vi "LaserMarked_ProjectSetPanel.vi"(11 "SetPanelRef":refnum<vi>) -> ()   [LabVIEW 2019]
uses:
  <vilib>/Utility/miscctls.llb/LVPointTypeDef.ctl
  <vilib>/Utility/miscctls.llb/LVPositionTypeDef.ctl
panel:
  out "$Read Project Recipe 2":path=path "C:/Users/MyUser/Desktop/S2_Project.txt" caption="讀取專案名稱路徑"
  in  "$Standar VNum_":string caption="電壓上限"
  in  "$NGY":i32 caption="料盤陣列Y" min=0 step=1
  in  "$NGX":i32 caption="料盤陣列X" min=0 step=1
  in  "$AIY":i32 caption="料盤AI拍照Y方向次數" min=0 step=1
  in  "$AIX":i32 caption="料盤AI拍照X方向次數" min=0 step=1
  in  "$LSY":i32 caption="料盤線掃瞄Y方向次數" min=0 step=1
  in  "$LSX":i32 caption="料盤線掃瞄X方向次數" min=0 step=1
  in  "$VISA resource name":refnum<visa-resource-name>
  in  "$VType":enum16{"無條件捨去", "四捨五入"}(ring) caption="電壓選取方式"
  in  "$Ring":u16(ring) caption="Ring" items=["A", "V", "C"]
  in  "Tab Control":enum32{"Page 1", "Page 2"}(tab)
  in  "$PLC_First PD No":i32 caption="PLC 使用首件號碼" min=0 step=1
  in  "$Read Tool Initial Project":path=path "C:/Users/MyUser/Desktop/S2_Project.txt" caption="讀取Tool Initial專案"
  in  "$Read S4 Tool Project":path=path "C:/Users/MyUser/Desktop/S2_Project.txt" caption="讀取S4 Tool專案路徑"
  in  "$Read S3 Tool Project":path=path "C:/Users/MyUser/Desktop/S2_Project.txt" caption="讀取S3 Tool專案路徑"
  in  "$Read S2 Tool Project":path=path "C:/Users/MyUser/Desktop/S2_Project.txt" caption="讀取S2 Tool專案路徑"
  in  "$RSSI Dn":dbl caption="RSSI下限" format="%#_13g"
  in  "$RSSI Up":dbl caption="RSSI上限" format="%#_13g"
  in  "$V Dn":dbl caption="V下限" format="%#_13g"
  in  "$C Dn":dbl caption="C(溫度值)下限" format="%#_13g"
  in  "$C Up":dbl caption="C(溫度值上限)" format="%#_13g"
  in  "$V Up":dbl caption="V 上限" format="%#_13g"
  in  "$MeasurLow":dbl caption="測高下限" format="%#_13g"
  in  "$MeasurHigh":dbl caption="測高上限" format="%#_13g"
  in  "$Current Dn":dbl caption="電流下限" format="%#_13g"
  in  "$Voltage Dn":dbl caption="電壓下限" format="%#_13g"
  in  "$ForceSetBinChk_":bool caption="使用參數確認"
  in  "$Voltage Up":dbl caption="電壓上限" format="%#_13g"
  in  "$Current Up":dbl caption="電流上限" format="%#_13g"
  in  "$PLC_Project No":i32 caption="PLC 使用專案號碼" min=0 step=1
  # "藍芽檢查參數設定"
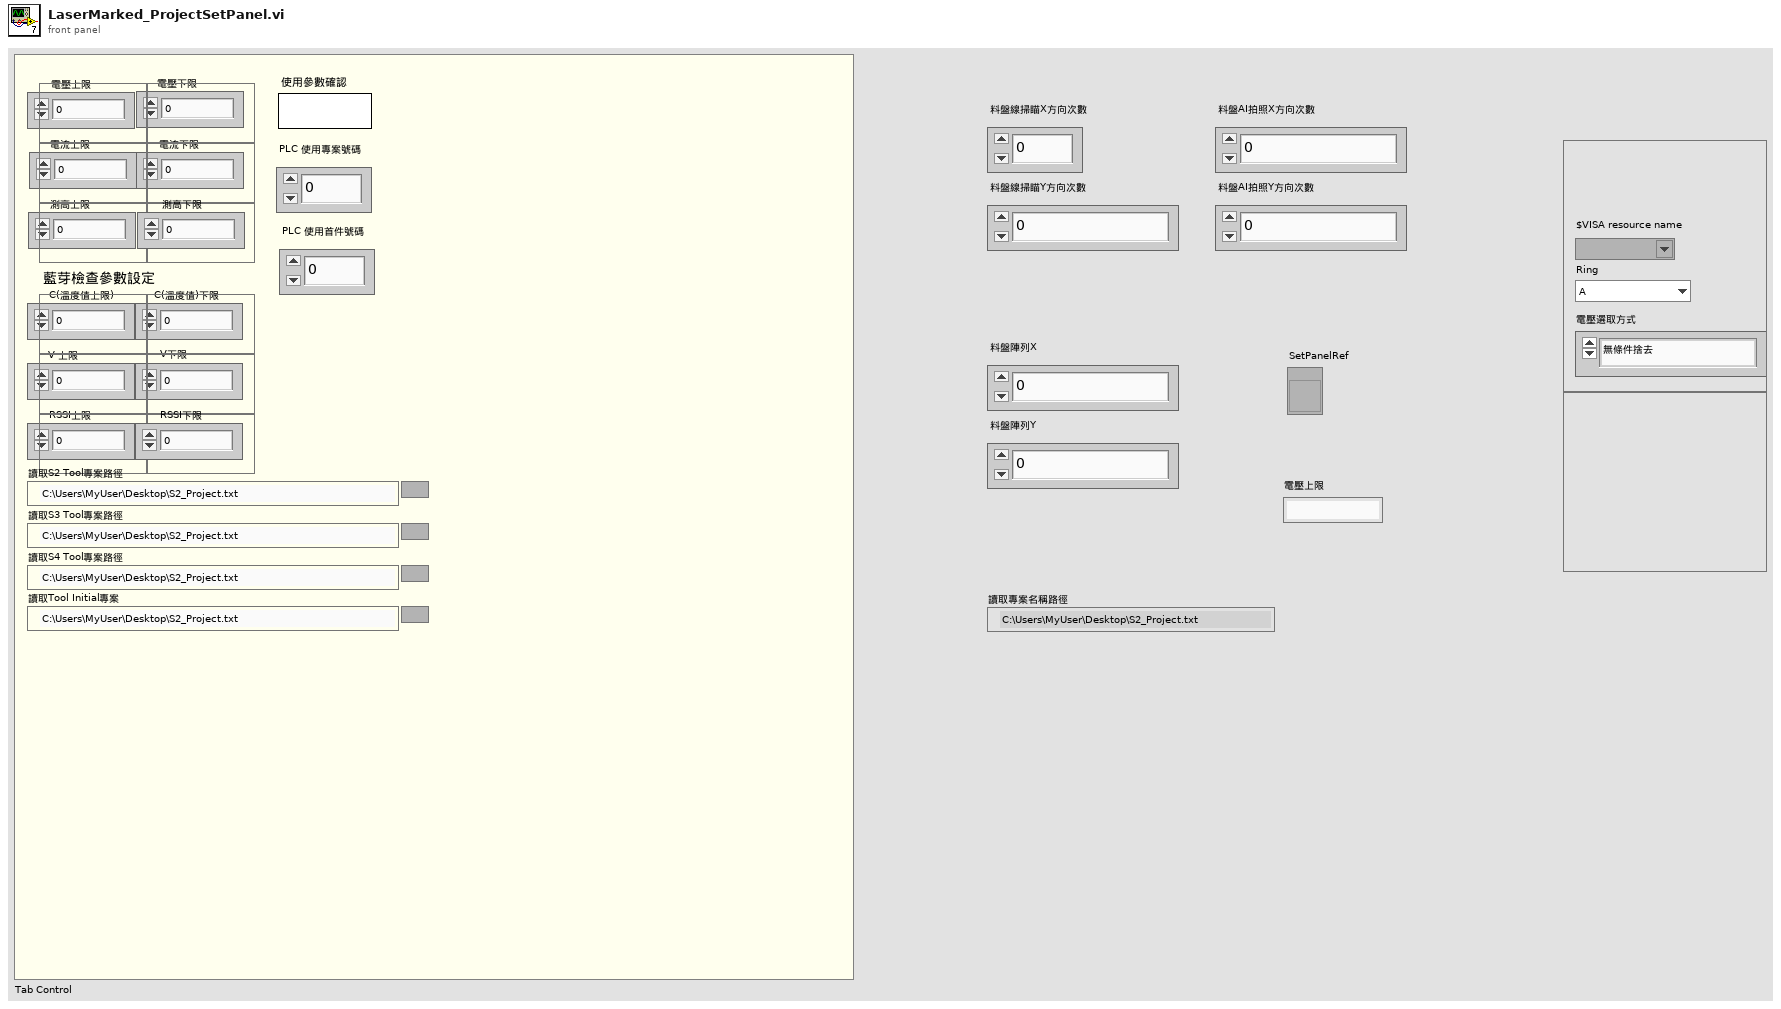
[diagram p1: front panel]
types:
  T1 = typedef "LVPositionTypeDef.ctl" = cluster{"Left":i32, "Top":i32}
  T2 = typedef "LVPointTypeDef.ctl" = cluster{"Horizontal":i16, "Vertical":i16}
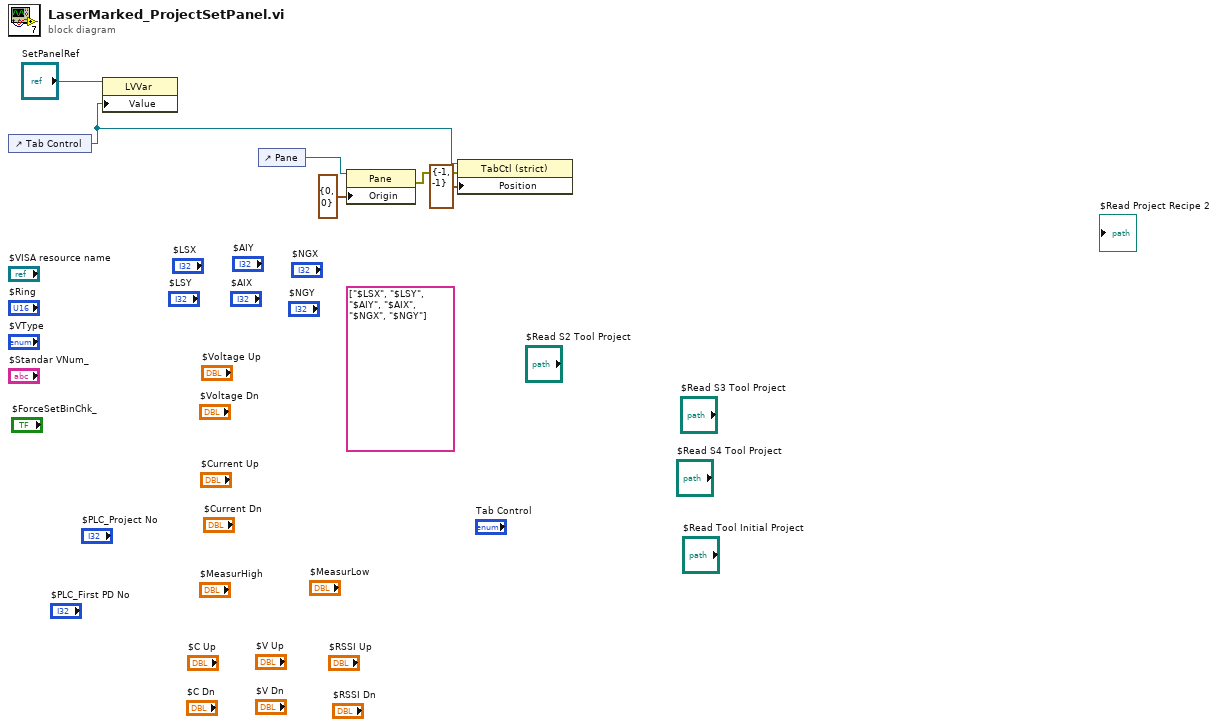
[diagram p0: block diagram]
diagram:
  (unwired) string[] ["$LSX", "$LSY", "$AIY", "$AIX", "$NGX", "$NGY"]
  n1 = control-ref of="Tab Control"() -> (w2:refnum<vi>)
  n2 = property class="LVVar"(reference="SetPanelRef", "Value"=w2) -> ()  [unwired: 1 in, 2 out]
  n3 = control-ref of="Pane"() -> (w5:refnum<vi>)
  n4 = property class="Pane"(reference=w5, "Origin"=T2 {"Horizontal"=0, "Vertical"=0}) -> (error out=w3:errorcluster)  [unwired: 1 in, 1 out]
  n5 = property class="TabCtl (strict)"(reference=w2, error in=w3, "Position"=T1 {"Left"=-1, "Top"=-1}) -> ()  [unwired: 2 out]
